vi "ENPH 354 Assignment 3 - Q3 .vi"() -> ()   [LabVIEW 2021]
panel:
  in  "?":bool
  out "Result Display":string
  in  "Cluster":T1
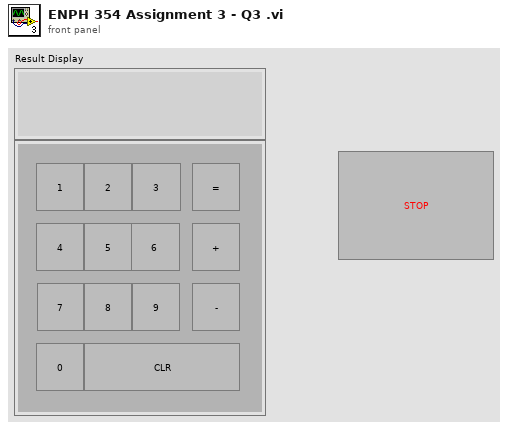
[diagram p1: front panel]
types:
  T1 = cluster{"4":bool, "-":bool, "+":bool, "CLR":bool, "=":bool, "6":bool, "7":bool, "8":bool, "9":bool, "2":bool, "3":bool, "5":bool, "1":bool, "0":bool}
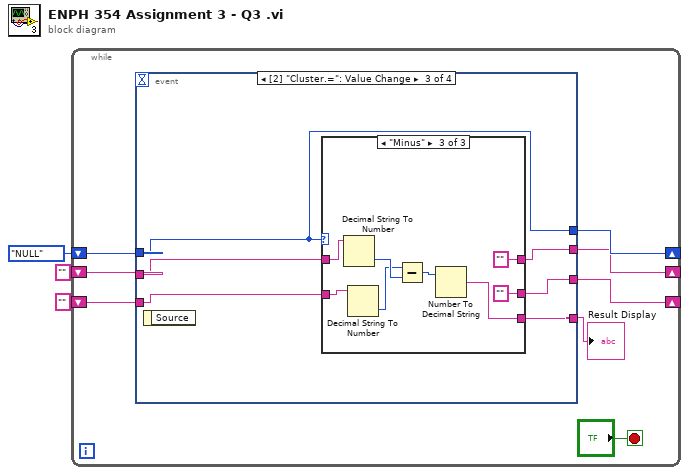
[diagram p0: block diagram]
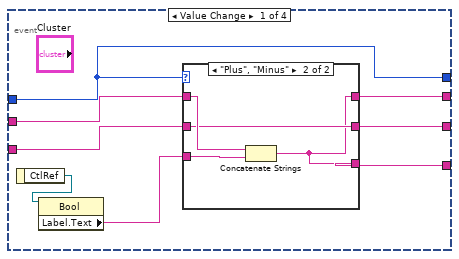
[diagram p2: hidden frame]
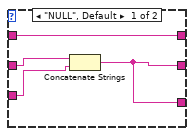
[diagram p3: hidden frame]
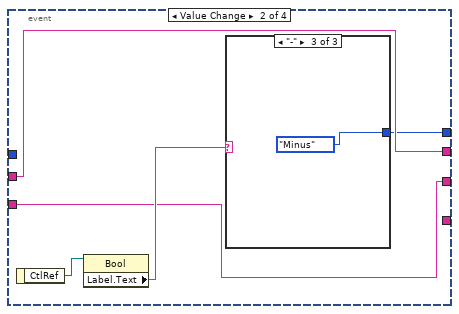
[diagram p4: hidden frame]
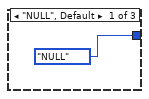
[diagram p5: hidden frame]
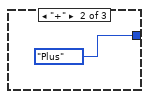
[diagram p6: hidden frame]
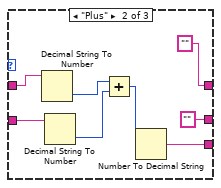
[diagram p8: hidden frame]
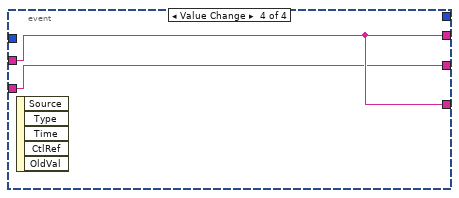
[diagram p9: hidden frame]
diagram:
  n1 = while {
    shift-right: [w9] -> _
    shift-left: enum16{"NULL", "Plus", "Minus"}."NULL" -> [w11]
    shift-right: [w6] -> _
    shift-left: "" -> [w7]
    shift-right: [w8] -> _
    shift-left: "" -> [w10]
    stop <- "?" stop-if-true
    n2 = event shown="[2] \"Cluster.=\": Value Change" {
      selector: _ -> [_ _ _ _]
      dyn-events: _ -> [_ _ _ _]
      timeout: _ -> [_ _ _ _]
      tunnel: w11 -> [w16 _ w41 _]
      tunnel: w10 -> [w17 w30 w39 w60]
      tunnel: [w16 w28 w41 _] -> w9
      tunnel: [w15 w30 w38 w60] -> w8
      tunnel: w7 -> [w14 w29 w40 w61]
      tunnel: [w13 w29 w37 w61] -> w6
      tunnel: [w12 _ w36 w61] -> w5
      event "Cluster.1", "Cluster.2", "Cluster.3", "Cluster.4", "Cluster.5", "Cluster.6", "Cluster.7", "Cluster.8", "Cluster.9", "Cluster.0": Value Change {
        n3 = event-data() -> ("CtlRef"=w19:refnum<vi>)  [unwired: 1 in]
        n4 = property class="Bool"(reference=w19) -> ("Label.Text"=w18:string)  [unwired: 1 in, 2 out]
        n5 = case shown="\"Plus\", \"Minus\"" w16 {
          tunnel: w18 -> [w23 w27]
          tunnel: w17 -> [w22 w25]
          tunnel: [w21 w25] -> w15
          tunnel: w14 -> [w20 w26]
          tunnel: [w20 w24] -> w13
          tunnel: [w21 w24] -> w12
          frame "NULL", Default {
            n6 = Concatenate Strings(w22, w23) -> (w21:string)
          }
          frame "Plus", "Minus" {
            n7 = Concatenate Strings(w26, w27) -> (w24:string)
          }
        }
      }
      event "Cluster.-", "Cluster.+": Value Change {
        n8 = event-data() -> ("CtlRef"=w32:refnum<vi>)  [unwired: 1 in]
        n9 = property class="Bool"(reference=w32) -> ("Label.Text"=w31:string)  [unwired: 1 in, 2 out]
        n10 = case shown="\"-\"" w31 {
          tunnel: [enum16{"NULL", "Plus", "Minus"}."NULL" enum16{"NULL", "Plus", "Minus"}."Plus" enum16{"NULL", "Plus", "Minus"}."Minus"] -> w28
          frame "NULL", Default {
          }
          frame "+" {
          }
          frame "-" {
          }
        }
      }
      event "Cluster.=": Value Change {
        n11 = event-data() -> ()  [unwired: 1 in, 1 out]
        n12 = case shown="\"Minus\"" w41 {
          tunnel: [w42 "" ""] -> w37
          tunnel: w40 -> [w42 w50 w58]
          tunnel: [w43 "" ""] -> w38
          tunnel: w39 -> [w43 w51 w59]
          tunnel: [w42 w46 w54] -> w36
          frame "NULL", Default {
          }
          frame "Plus" {
            n13 = Decimal String To Number(string=w50) -> (number=w49:i32)  [unwired: 2 in, 1 out]
            n14 = Decimal String To Number(string=w51) -> (number=w48:i32)  [unwired: 2 in, 1 out]
            n15 = Add(x=w49, y=w48) -> (x+y=w47:i32)
            n16 = Number To Decimal String(number=w47) -> (decimal integer string=w46:string)  [unwired: 1 in]
          }
          frame "Minus" {
            n17 = Decimal String To Number(string=w58) -> (number=w53:i32)  [unwired: 2 in, 1 out]
            n18 = Decimal String To Number(string=w59) -> (number=w52:i32)  [unwired: 2 in, 1 out]
            n19 = Subtract(x=w52, y=w53) -> (x-y=w57:i32)
            n20 = Number To Decimal String(number=w57) -> (decimal integer string=w54:string)  [unwired: 1 in]
          }
        }
      }
      event "Cluster.CLR": Value Change {
        n21 = event-data() -> ()  [unwired: 1 in, 5 out]
      }
    }
    "Result Display" <- w5
  }
